vi "VI Tree.vi"   [LabVIEW 2012, in "Phidget GPS.lvlib"]
doc: "${GPS:VITreeHeader}"
uses:
  <instrlib>/Phidgets/Phidget GPS/Phidget GPS.lvlib
  <instrlib>/Phidgets/Phidget GPS/Public/GPSStart.vi
  <instrlib>/Phidgets/Phidget GPS/Public/GPSOpen.vi
  <instrlib>/Phidgets/Phidget GPS/Public/GPSClose.vi
panel:
  # "(c) 2015 Phidgets Inc..  ALL RIGHTS RESERVED."
  # "SEE DIAGRAM\nFOR VI TREE."
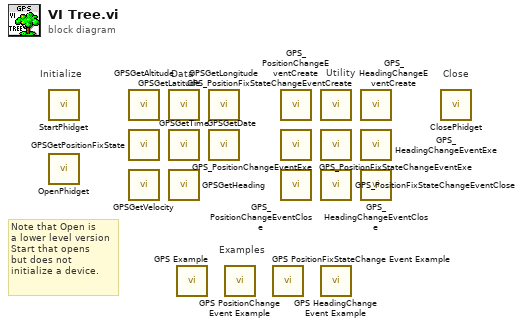
[diagram p0: block diagram]
diagram:
  # "Note that Open is\na lower level version\nStart that opens\nbut does not \ninitialize a device."
  # "Examples"
  # "Utility"
  # "Data"
  # "Close"
  # "Initialize"
  n1 = call-poly <instrlib>:"StartPhidget.vi"() -> ()  [unwired: 12 in, 4 out]
  n2 = call-poly <instrlib>:"OpenPhidget.vi"() -> ()  [unwired: 8 in, 4 out]
  n3 = call <instrlib>:"GPSGetAltitude.vi"() -> ()  [unwired: 8 in, 3 out]
  n4 = call <instrlib>:"GPSGetPositionFixState.vi"() -> ()  [unwired: 8 in, 3 out]
  n5 = call <instrlib>:"GPSGetVelocity.vi"() -> ()  [unwired: 8 in, 3 out]
  n6 = call <instrlib>:"GPSGetLatitude.vi"() -> ()  [unwired: 8 in, 3 out]
  n7 = call <instrlib>:"GPSGetTime.vi"() -> ()  [unwired: 8 in, 3 out]
  n8 = call <instrlib>:"GPSGetHeading.vi"() -> ()  [unwired: 8 in, 3 out]
  n9 = call <instrlib>:"GPS Example.vi"() -> ()  [unwired: 12 in]
  n10 = call <instrlib>:"GPSGetLongitude.vi"() -> ()  [unwired: 8 in, 3 out]
  n11 = call <instrlib>:"GPSGetDate.vi"() -> ()  [unwired: 8 in, 3 out]
  n12 = call <instrlib>:"GPS PositionChange Event Example.vi"() -> ()  [unwired: 12 in]
  n13 = call <instrlib>:"GPS PositionFixStateChange Event Example.vi"() -> ()  [unwired: 12 in]
  n14 = call <instrlib>:"GPS_PositionChangeEventCreate.vi"() -> ()  [unwired: 9 in, 3 out]
  n15 = call <instrlib>:"GPS_PositionChangeEventExe.vi"() -> ()  [unwired: 11 in, 9 out]
  n16 = call <instrlib>:"GPS_PositionChangeEventClose.vi"() -> ()  [unwired: 10 in, 2 out]
  n17 = call <instrlib>:"GPS_PositionFixStateChangeEventCreate.vi"() -> ()  [unwired: 9 in, 3 out]
  n18 = call <instrlib>:"GPS_PositionFixStateChangeEventExe.vi"() -> ()  [unwired: 5 in, 7 out]
  n19 = call <instrlib>:"GPS_PositionFixStateChangeEventClose.vi"() -> ()  [unwired: 10 in, 2 out]
  n20 = call <instrlib>:"GPS HeadingChange Event Example.vi"() -> ()  [unwired: 12 in]
  n21 = call <instrlib>:"GPS_HeadingChangeEventCreate.vi"() -> ()  [unwired: 9 in, 3 out]
  n22 = call <instrlib>:"GPS_HeadingChangeEventExe.vi"() -> ()  [unwired: 8 in, 8 out]
  n23 = call <instrlib>:"GPS_HeadingChangeEventClose.vi"() -> ()  [unwired: 10 in, 2 out]
  n24 = call-poly <instrlib>:"ClosePhidget.vi"() -> ()  [unwired: 11 in, 1 out]
